vi "Tutorial 1_temperature.vi"() -> ()   [LabVIEW 2020]
panel:
  in  "Thermometer C":dbl(slide) scale=0.0..100.0
  out "mode":string
  out "Temp":dbl
  out "Warning Alam":bool
  in  "Switch":bool
  out "output control":dbl
  in  "input control":dbl
  # "input"
  # "output"
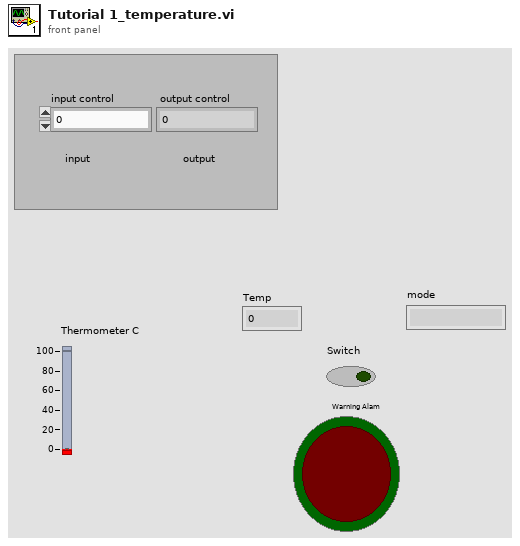
[diagram p1: front panel]
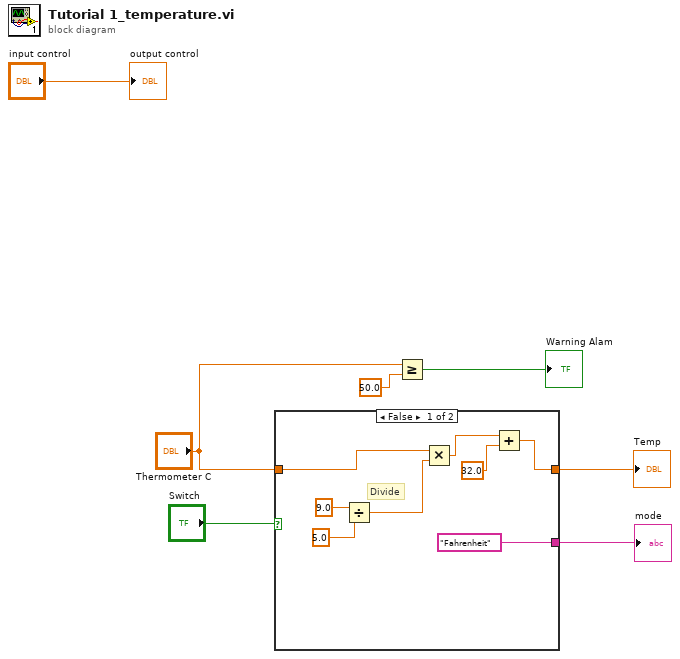
[diagram p0: block diagram]
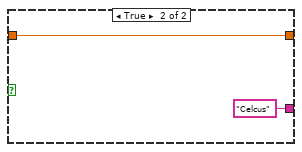
[diagram p2: hidden frame]
diagram:
  n1 = case shown="False" "Switch" {
    tunnel: [w9 w17] -> w5
    tunnel: "Thermometer C" -> [w13 w17]
    tunnel: ["Fahrenheit" ("mode") "Celcus" ("mode")] -> w4
    frame False {
      # "Divide"
      n2 = Divide(x=9.0, y=5.0) -> (x/y=w11:dbl)
      n3 = Multiply(x=w13, y=w11) -> (x*y=w10:dbl)
      n4 = Add(x=w10, y=32.0) -> (x+y=w9:dbl)
    }
    frame True {
    }
  }
  "Temp" <- w5
  "mode" <- w4
  n5 = Greater Or Equal?(x="Thermometer C", y=50.0) -> (x >= y?=→"Warning Alam":bool)
  "output control" <- "input control"
